vi "WorkorderHandler_New.vi"(2 "data":T2, 5 "error in (no error)":errorcluster, 8 "object name (unnamed)":string) -> (14 "reference":T1, 19 "error out":errorcluster)   [LabVIEW 2011]
doc: "Creates new dqGOOP object and returns a refnum"
uses:
  DataStructures/WorkorderHandler_ObjectData.ctl
  DataStructures/WorkorderHandler_ObjectReference.ctl
panel:
  in  "reference (default)":T1
  # "Copyright (C) 2004 DataAct Incorporated"
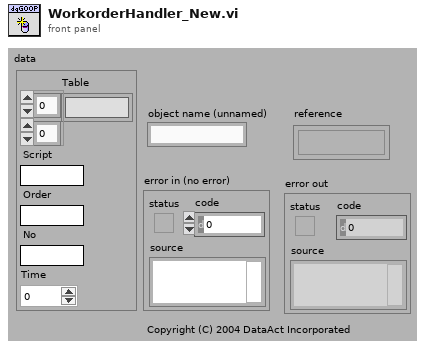
[diagram p1: front panel]
types:
  T1 = typedef "WorkorderHandler_ObjectReference.ctl" = refnum<k1>
  T2 = typedef "WorkorderHandler_ObjectData.ctl" = cluster{"Table":string[][], "Script":string, "Order":string, "No":string, "Time":dbl}
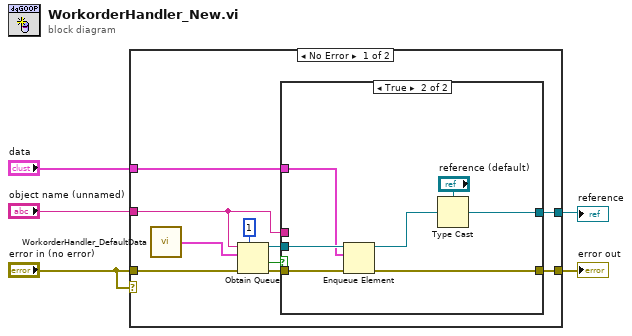
[diagram p0: block diagram]
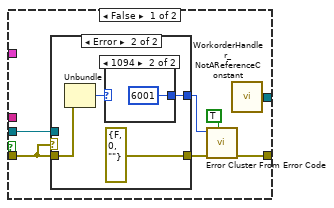
[diagram p2: hidden frame]
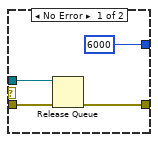
[diagram p3: hidden frame]
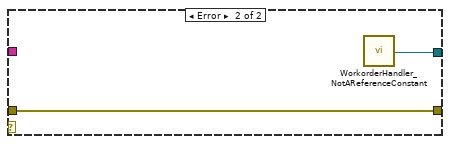
[diagram p5: hidden frame]
diagram:
  n1 = case shown="No Error" "error in (no error)" {
    tunnel: [w11 w40] -> w5
    tunnel: [w9 w41] -> w4
    tunnel: "error in (no error)" -> [w8 w40]
    tunnel: "object name (unnamed)" -> [w7 _]
    tunnel: "data" -> [w6 _]
    frame No Error {
      n2 = call "WorkorderHandler_DefaultData.vi"() -> ("data"=w10:T2)
      n3 = Obtain Queue(max queue size (-1, unlimited)=1, name (unnamed)=w7, element data type=w10, error in (no error)=w8) -> (queue out=w15:refnum<queue>, created new?=w12:bool, error out=w14:errorcluster)  [unwired: 1 in]
      n4 = case shown="True" w12 {
        tunnel: w15 -> [w22 w39]
        tunnel: w14 -> [w20 w38]
        tunnel: [w18 w37] -> w11
        tunnel: w7 -> [_ _]
        tunnel: [w21 w34] -> w9
        tunnel: w6 -> [_ w36]
        frame False {
          n5 = case shown="Error" w20 {
            tunnel: w20 -> [w26 w28]
            tunnel: w22 -> [w25 _]
            tunnel: [w24 errorcluster {"status"=FALSE, "code"=0, "source"=""} ("error out")] -> w19
            tunnel: [6000 ("code") w29] -> w16
            frame No Error {
              n6 = Release Queue(queue=w25, error in (no error)=w26) -> (error out=w24:errorcluster)  [unwired: 3 out]
            }
            frame Error {
              n7 = Unbundle(w28) -> ("code"=w30:i32)  [unwired: 2 out]
              n8 = case shown="1094" w30 {
                selector: w30 -> [w31 _]
                tunnel: [w31 6001 ("code")] -> w29
                frame Default {
                }
                frame 1094 {
                }
              }
            }
          }
          n9 = call <vilib>:"Error Cluster From Error Code.vi"("show call chain? (False)"=TRUE, "error in (no error)"=w19, "error code (0)"=w16) -> ("error out"=w18:errorcluster)  [unwired: 6 out]
          n10 = call "WorkorderHandler_NotAReferenceConstant.vi"() -> ("reference"=w21:T1)
        }
        frame True {
          n11 = Enqueue Element(queue=w39, element=w36, error in (no error)=w38) -> (queue out=w33:refnum<queue>, error out=w37:errorcluster)  [unwired: 2 out]
          n12 = Type Cast(type="reference (default)", x=w33) -> (*(type *) &x=w34:T1)
        }
      }
    }
    frame Error {
      n13 = call "WorkorderHandler_NotAReferenceConstant.vi"() -> ("reference"=w41:T1)
    }
  }
  "error out" <- w5
  "reference" <- w4
